vi "New Resource from ANSI Item.vi"(7 "Shared? (f)":bool, 8 "error in (no error)":errorcluster, 9 "Default String (ANSI)":string, 10 "Tag (ANSI)":string, 11 "LangFile in":refnum<class "Resource Data.lvclass">) -> (0 "error out":errorcluster, 2 "RID":string, 3 "LangFile out":refnum<class "Resource Data.lvclass">)   [LabVIEW 2013, in "SET Project Data.lvlib" / "Resource Data.lvclass"]
uses:
  Resource Data.lvclass
  Types/ProjFile_Resource Entry.ctl
  Resource Data.lvclass/Resource Data.ctl
  Read Languages.vi
  SET Project Data.lvlib
  Lib/Unicode/SET_Unicode Tools.lvlib
panel:
  # "- Convert strings to unicode\n- Generate new RID\n- Add entry to resource table"
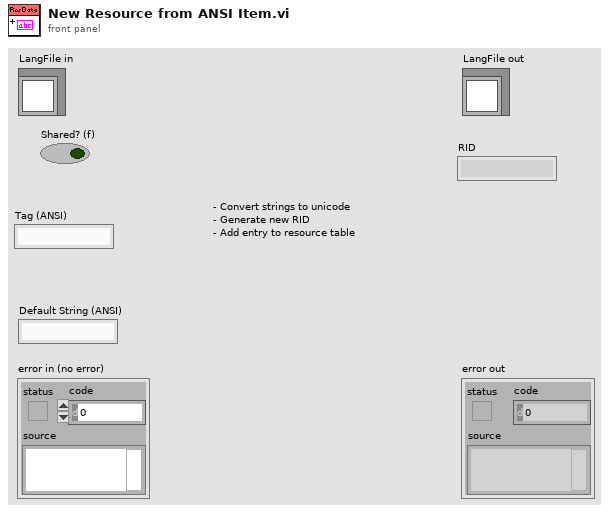
[diagram p1: front panel]
types:
  T1 = typedef "SET Project Data.lvlib/ProjFile_Resource Entry.ctl" = cluster{"RID":string, "Tag":string, "Strings [] (UTF-16)":string[], "Shared?":bool}
  T2 = typedef "SET Project Data.lvlib/ProjFile_Language Data.ctl" = cluster{"Tag":string, "Name":string, "Code Page":u16}
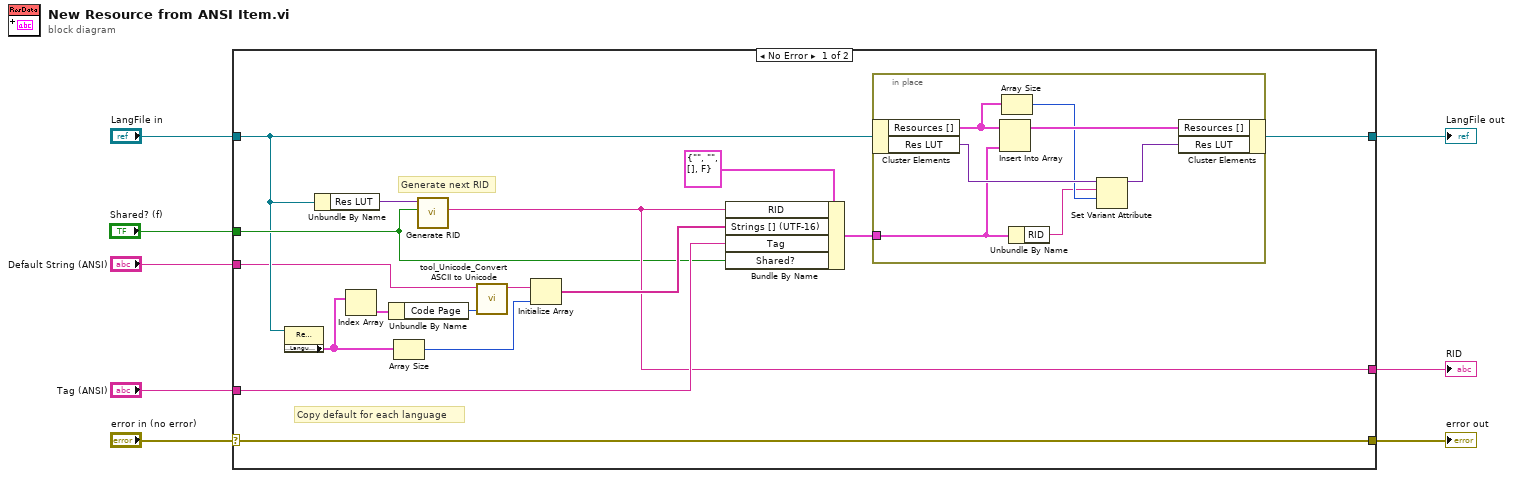
[diagram p0: block diagram]
diagram:
  n1 = case shown="No Error" "error in (no error)" {
    selector: "error in (no error)" -> [w24 w33]
    tunnel: [w24 w33] -> w7
    tunnel: [w21 w32] -> w5
    tunnel: "LangFile in" -> [w14 w32]
    tunnel: "Shared? (f)" -> [w15 _]
    tunnel: "Tag (ANSI)" -> [w18 _]
    tunnel: "Default String (ANSI)" -> [w11 _]
    tunnel: [w16 _] -> w1
    frame No Error {
      # "Copy default for each language"
      # "Generate next RID"
      n2 = property class="Resource Data.lvclass"(reference=w14) -> ("Properties:Languages []"=w13:T2[])  [unwired: 1 in, 2 out]
      n3 = Unbundle By Name(w14) -> ("Res LUT"=w17:variant)
      n4 = Index Array(array=w13) -> (element=w12:T2)  [unwired: 1 in]
      n5 = Unbundle By Name(w12) -> ("Code Page"=w9:u16)
      n6 = Array Size(array=w13) -> (size(s)=w23:i32)
      n7 = call "Generate RID.vi"("Negative? (F)"=w15, "LUT in"=w17) -> ("Unique Key"=w16:string)  [unwired: 8 in, 1 out]
      n8 = call "tool_Unicode_Convert ASCII to Unicode.vi"("Source Code Page"=w9, "MultiByteStr (ANSI)"=w11) -> ("WideCharStr (UTF-16LE)"=w10:string)  [unwired: 8 in, 1 out]
      n9 = Initialize Array(w10, w23) -> (w19:string[])
      n10 = Bundle By Name(cluster=T1 {"RID"="", "Tag"="", "Strings [] (UTF-16)"=[], "Shared?"=FALSE} ("Resource"), "RID"=w16, "Strings [] (UTF-16)"=w19, "Tag"=w18, "Shared?"=w15) -> (w20:T1)
      n11 = in-place {
        in-place-border: w20 -> [w26]
        n12 = in-place-cluster #1(w14) -> ("Resources []"=w28:T1[], "Res LUT"=w30:variant)
        n13 = Insert Into Array(array=w28, new element=w26) -> (w31:T1[])  [unwired: 1 in]
        n14 = Array Size(array=w28) -> (size(s)=w27:i32)
        n15 = Unbundle By Name(w26) -> ("RID"=w25:string)
        n16 = Set Variant Attribute(Variant=w30, name=w25, value=w27) -> (Variant out=w29:variant)  [unwired: 1 in, 2 out]
        n17 = in-place-cluster #1("Resources []"=w31, "Res LUT"=w29) -> (w21:refnum<class "Resource Data.lvclass">)
      }
    }
    frame Error {
    }
  }
  "error out" <- w7
  "LangFile out" <- w5
  "RID" <- w1
